vi "Draw Arrow Line.vi"(6 "Draw Para":T1={"fill?(F)"=TRUE, "color(black)"=0, "pen"={"Width"=1, "Style"=enum."Solid"}}, 8 "错误输入":errorcluster, 9 "Arrow":T2={"Line Len"=20, "Arrow dx"=-5, "Arrow dy"=5, "Line Angle"=0.0}, 10 "Start Pointx,y)":cluster{"x":i16, "y":i16} caption="Start Point(x,y)", 11 "Pic in":picture) -> (0 "错误输出":errorcluster, 3 "Pic out":picture)   [LabVIEW 2012, in "Picture Box Tools.lvlib" / "Basic Shape.lvlib"]
uses:
  Basic Shape.lvlib
  Draw Para Custom Control.ctl
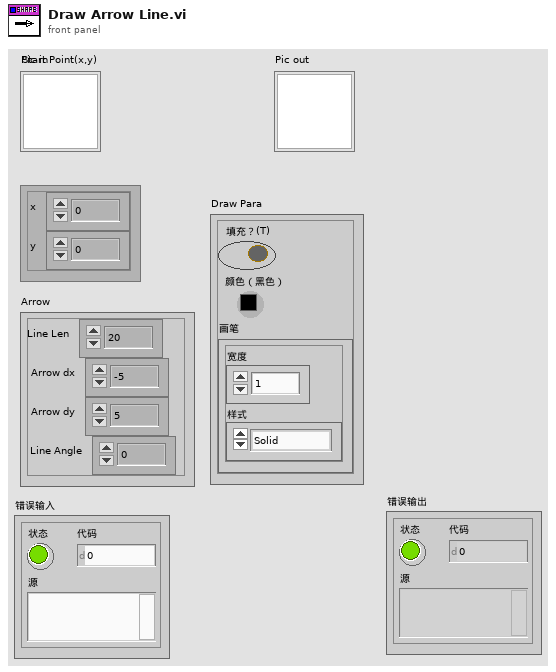
[diagram p1: front panel]
types:
  T1 = typedef "Picture Box Tools.lvlib/Basic Shape.lvlib/Draw Para Custom Control.ctl" = cluster{"fill?(F)":bool, "color(black)":u32, "pen":cluster{"Width":u16, "Style":enum32{"Solid", "Dash", "Dot", "DashDot", "DashDotDot"}}}
  T2 = cluster{"Line Len":i16, "Arrow dx":i16, "Arrow dy":i16, "Line Angle":dbl}
  T3 = cluster{"Width":u16, "Style":enum32{"Solid", "Dash", "Dot", "DashDot", "DashDotDot"}}
  T4 = typedef "Picture Box Tools.lvlib/Basic Shape.lvlib/Point Custom Control.ctl" = cluster{"horizontal":i16, "vertical":i16}
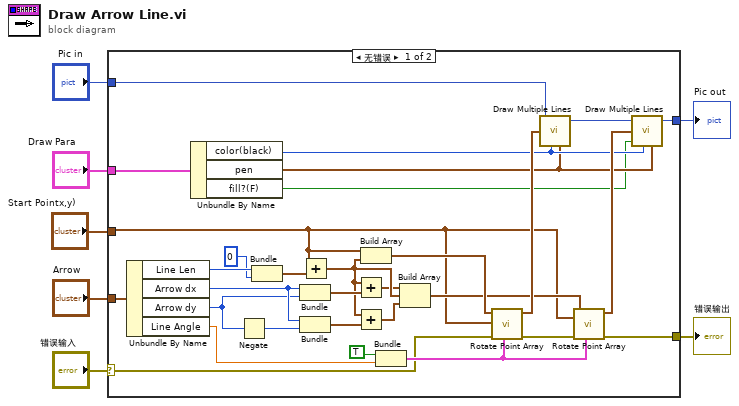
[diagram p0: block diagram]
diagram:
  n1 = case shown="无错误" "错误输入" {
    selector: "错误输入" -> [w20 w38]
    tunnel: [w18 w38] -> w6
    tunnel: "Arrow" -> [w17 _]
    tunnel: "Start Pointx,y)" -> [w16 _]
    tunnel: "Pic in" -> [w15 w39]
    tunnel: [w14 w39] -> w2
    tunnel: "Draw Para" -> [w13 _]
    frame No Error {
      n2 = Unbundle By Name(w17) -> ("Line Len"=w37:i16, "Arrow dx"=w33:i16, "Arrow dy"=w31:i16, "Line Angle"=w28:dbl)
      n3 = Unbundle By Name(w13) -> ("color(black)"=w12:u32, "pen"=w11:T3, "fill?(F)"=w8:bool)
      n4 = Negate(x=w31) -> (-x=w32:i16)
      n5 = Bundle("Line Len"=w37, "Line Len"=i16 0) -> (w35:cluster{"Line Len":i16, "Line Len":i16})  [unwired: 1 in]
      n6 = Bundle("Arrow dx"=w33, "Arrow dy"=w31) -> (w34:cluster{"Arrow dx":i16, "Arrow dy":i16})  [unwired: 1 in]
      n7 = Bundle("Arrow dx"=w33, w32) -> (w30:cluster{"Arrow dx":i16, i16})  [unwired: 1 in]
      n8 = Add(x=w16, y=w35) -> (x+y=w10:cluster{i16, i16})
      n9 = Add(x=w10, y=w34) -> (x+y=w9:cluster{i16, i16})
      n10 = Add(x=w10, y=w30) -> (x+y=w25:cluster{i16, i16})
      n11 = Build Array(w16, w10) -> (w27:cluster{"x":i16, "y":i16}[])
      n12 = Bundle("Absolute?"=TRUE, "Line Angle"=w28) -> (w21:cluster{"Absolute?":bool, "Line Angle":dbl})  [unwired: 1 in]
      n13 = Build Array(w9, w10, w25) -> (w24:cluster{i16, i16}[])
      n14 = call "Rotate Point Array.vi"("Para"=w21, "错误输入"=w20, "Center"=w16, "Point Array"=w27) -> ("错误输出"=w19:errorcluster, "Rotated Absolute Point Array"=w26:T4[])  [unwired: 5 in, 1 out]
      n15 = call <vilib>:"Draw Multiple Lines.vi"("picture"=w15, "line endpoints"=w26, "color(black)"=w12, "pen"=w11) -> ("new picture"=w22:picture)  [unwired: 5 in]
      n16 = call "Rotate Point Array.vi"("Para"=w21, "错误输入"=w19, "Center"=w16, "Point Array"=w24) -> ("错误输出"=w18:errorcluster, "Rotated Absolute Point Array"=w23:T4[])  [unwired: 5 in, 1 out]
      n17 = call <vilib>:"Draw Multiple Lines.vi"("picture"=w22, "line endpoints"=w23, "fill?(F)"=w8, "color(black)"=w12, "pen"=w11) -> ("new picture"=w14:picture)  [unwired: 4 in]
    }
    frame Error {
    }
  }
  "错误输出" <- w6
  "Pic out" <- w2
